vi "File Start.vi"(5 "Run in Background":bool=TRUE, 7 "Write Period":u32=3000, 8 "Error In":errorcluster) -> (0 "Error Out":errorcluster)   [LabVIEW 2018, in "Toolkit.lvlib"]
doc: "Starts writing logging statements to the default log file."
uses:
  Toolkit.lvlib
  Support/File/Action.ctl
  Support/File/File.lvlib
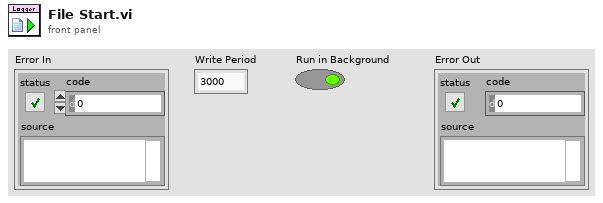
[diagram p1: front panel]
types:
  T1 = typedef "Toolkit.lvlib/File.lvlib/Action.ctl" = enum16{"Initialize", "Set Maximum File Size", "Set Maximum File Count", "Set Root Folder", "Set Enable Calendar Folder Tree", "Set File Extension", "Set Prune All", "Start", "Write", "Stop", "Shutdown"}
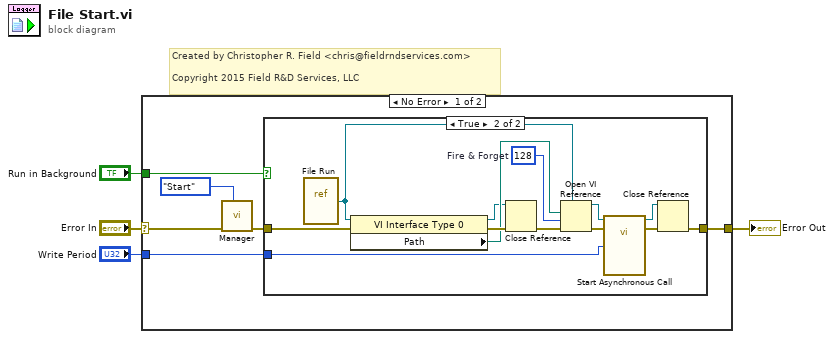
[diagram p0: block diagram]
diagram:
  # "Created by Christopher R. Field <chris@fieldrndservices.com>\n\nCopyright 2015 Field R&D Services, LLC"
  n1 = case shown="No Error" "Error In" {
    selector: "Error In" -> [w8 w25]
    tunnel: [w10 w25] -> w3
    tunnel: "Write Period" -> [w5 _]
    tunnel: "Run in Background" -> [w6 _]
    frame No Error {
      n2 = call "Manager.vi"("Action"=Action."Start", "Error In"=w8) -> ("Error Out"=w7:errorcluster)  [unwired: 9 in]
      n3 = case shown="True" w6 {
        tunnel: [w11 w14] -> w10
        tunnel: w7 -> [w11 w20]
        tunnel: w5 -> [_ w16]
        frame False {
        }
        frame True {
          w12 = 128  # Fire & Forget
          n4 = vi-ref "File Run.vi"() -> (w17:refnum<vi>)
          n5 = property class="VI Interface Type 0"(reference=w17, error in=w20) -> (reference out=w21:refnum<vi>, error out=w24:errorcluster, "Path"=w23:path)
          n6 = Close Reference(reference=w21, error in (no error)=w24) -> (error out=w22:errorcluster)
          n7 = Open VI Reference(type specifier VI Refnum (for type only)=w17, vi path=w23, options=w12, error in (no error)=w22) -> (vi reference=w18:refnum<vi>, error out=w19:errorcluster)  [unwired: 2 in]
          n8 = call-by-ref "Start Asynchronous Call"(reference=w18, error in=w19, "Write Period"=w16) -> (reference out=w13:refnum<vi>, error out=w15:errorcluster)  [unwired: 10 in, 1 out]
          n9 = Close Reference(reference=w13, error in (no error)=w15) -> (error out=w14:errorcluster)
        }
      }
    }
    frame Error {
    }
  }
  "Error Out" <- w3
